vi "string to system.vi"(8 "error in":errorcluster, 10 "targets to load (all)":string[](array[string]), 11 "data":string) -> (0 "error out":errorcluster, 2 "system":T1)   [LabVIEW 2013, in "PLConfigurationSerializer.lvlib"]
uses:
  PLConfigurationSerializer.lvlib
  systems cluster.ctl
  system configuration/PL_System Configuration.lvclass
  targets cluster.ctl
  target configuration/PL_Target Configuration.lvclass
  engines cluster.ctl
  <vilib>/NI/Module Execution Interface/Engine Configuration/engine configuration.lvclass
  <vilib>/NI/Tag Bus Module Framework/module configuration/TBM module configuration.lvclass
  targetlist.ctl
  enginelist.ctl
  modulelist.ctl
  class discovery singleton methods.ctl
  <vilib>/NI/Tag Bus Module Framework/root configuration/TBM configuration.lvclass
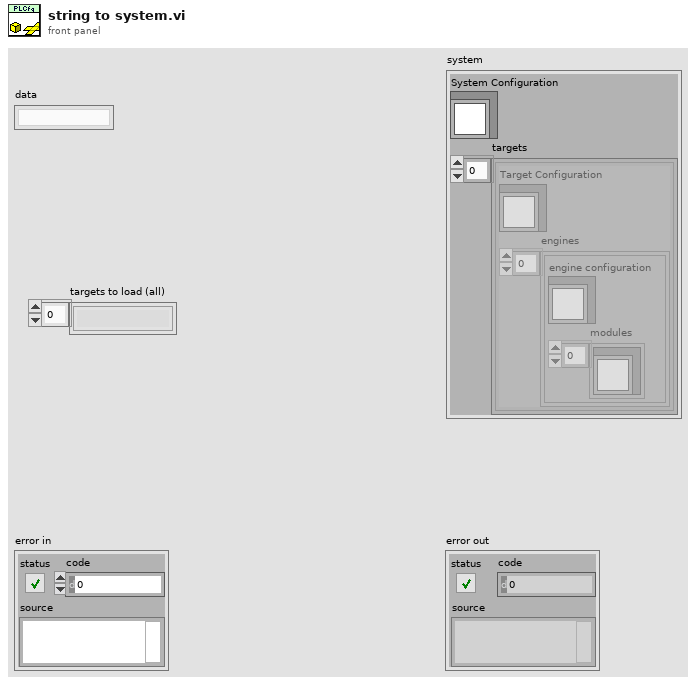
[diagram p1: front panel]
types:
  T1 = typedef "PLConfigurationSerializer.lvlib/systems cluster.ctl" = cluster{"System Configuration":refnum<class "PL_System Configuration.lvclass">, "targets":T2[]}
  T2 = typedef "PLConfigurationSerializer.lvlib/targets cluster.ctl" = cluster{"Target Configuration":refnum<class "PL_Target Configuration.lvclass">, "engines":T3[]}
  T3 = typedef "PLConfigurationSerializer.lvlib/engines cluster.ctl" = cluster{"engine configuration":refnum<class "engine configuration.lvclass">, "modules":refnum<class "TBM module configuration.lvclass">[]}
  T4 = typedef "PLConfigurationSerializer.lvlib/targetlist.ctl" = cluster{"name":string, "instanceid":string}
  T5 = typedef "PLConfigurationSerializer.lvlib/enginelist.ctl" = cluster{"engineid":string, "classname":string}
  T6 = typedef "PLConfigurationSerializer.lvlib/class discovery singleton methods.ctl" = enum16{"add search paths", "load class by name"}
  T7 = typedef "PLConfigurationSerializer.lvlib/modulelist.ctl" = cluster{"moduleid":string, "classname":string}
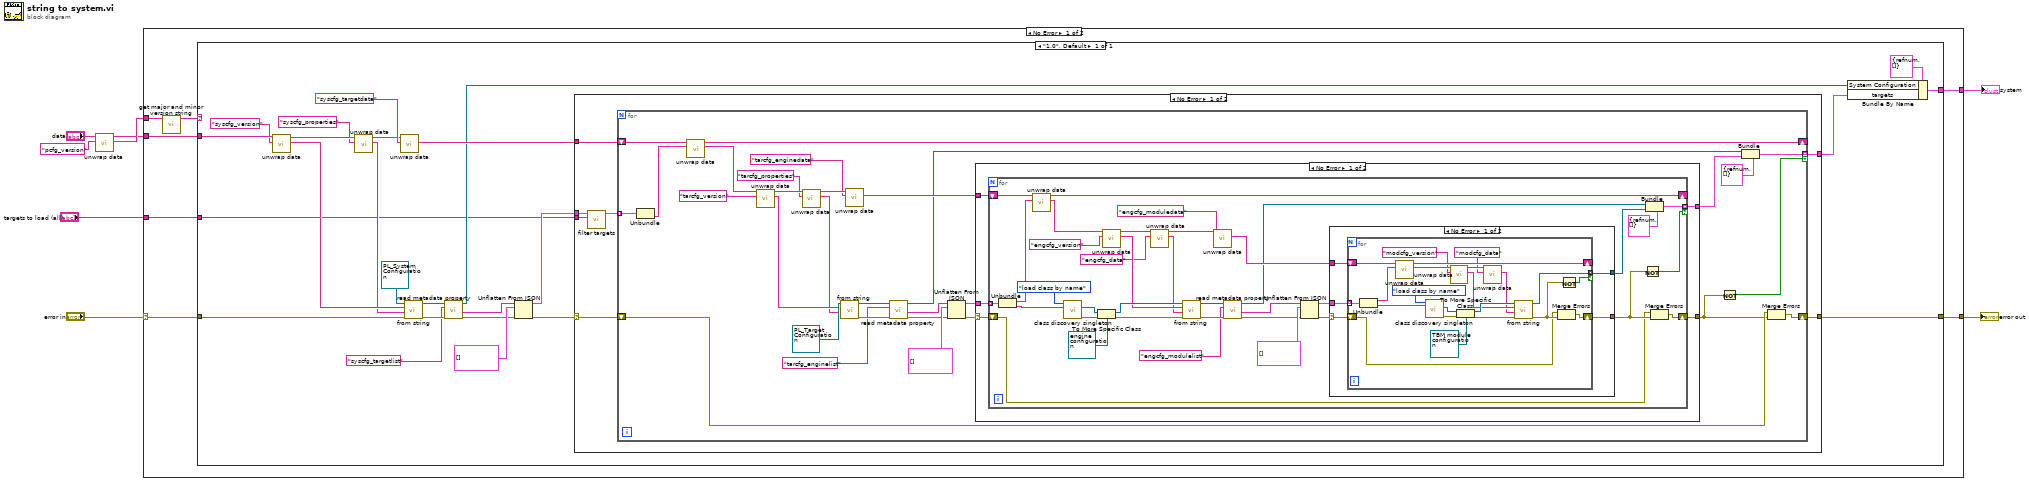
[diagram p0: block diagram]
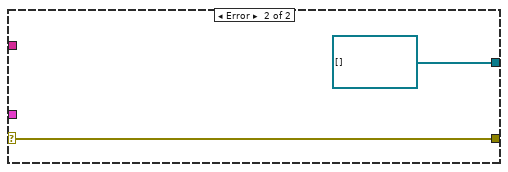
[diagram p2: hidden frame]
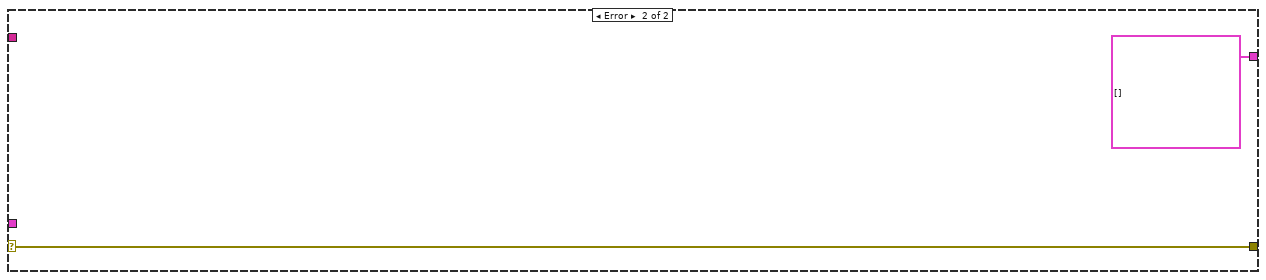
[diagram p3: hidden frame]
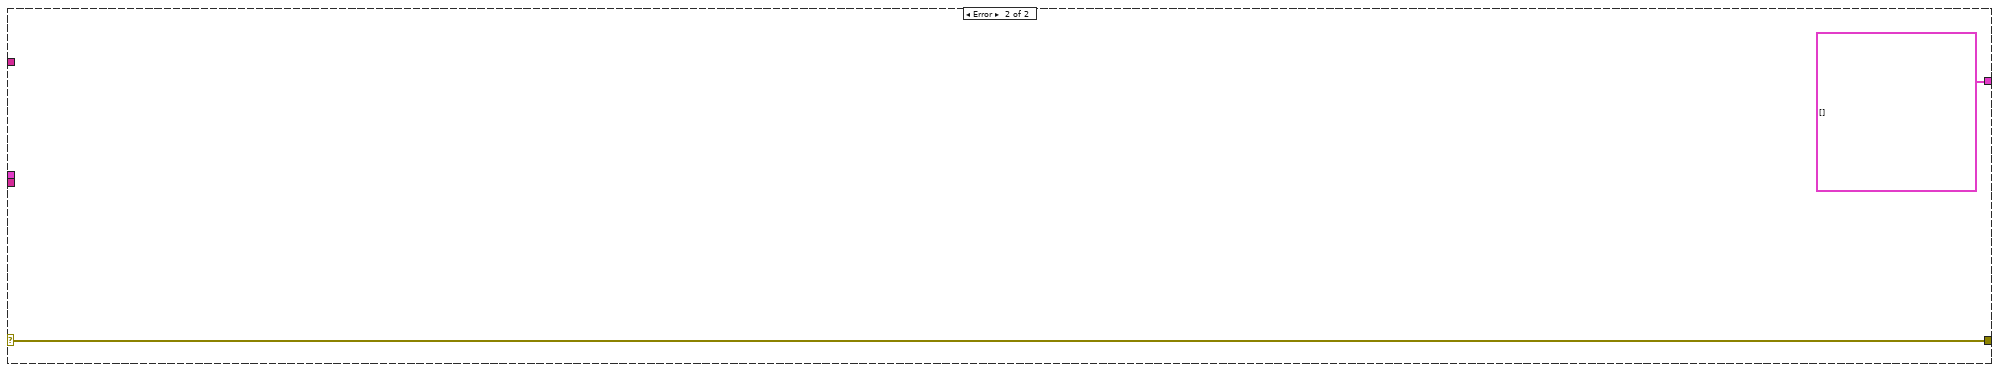
[diagram p4: hidden frame]
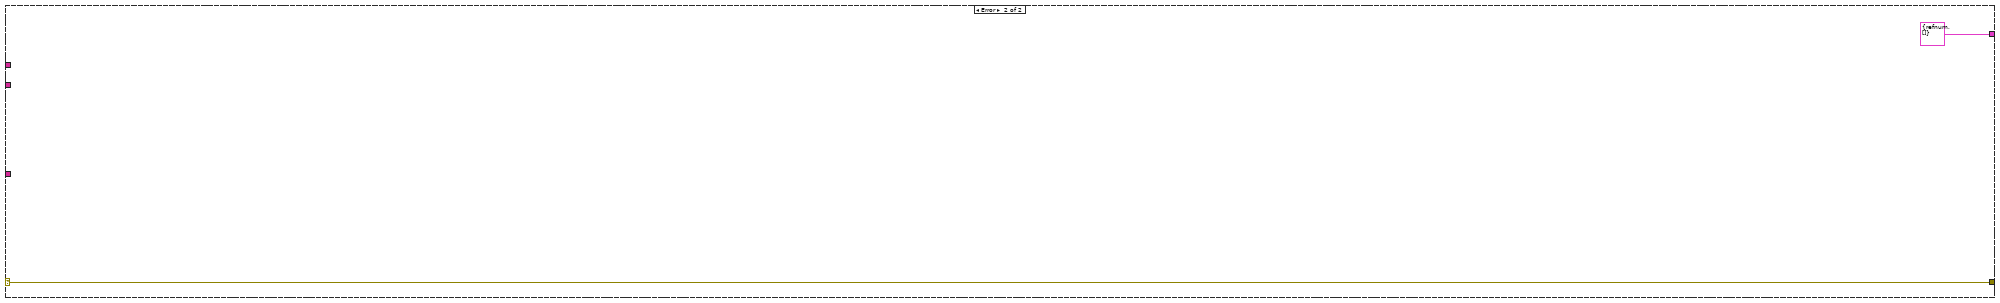
[diagram p5: hidden frame]
diagram:
  n1 = call <vilib>:"unwrap data.vi"("identifier"="pcfg_version" ("additional identifier"), "data to unwrap"="data") -> ("unwrapped data"=w7:string, "remaining string"=w6:string)  [unwired: 8 in]
  n2 = case shown="No Error" "error in" {
    selector: "error in" -> [w11 w153]
    tunnel: w6 -> [w15 _]
    tunnel: [w14 T1 {"System Configuration"=refnum, "targets"=[]} ("system")] -> w5
    tunnel: [w10 w153] -> w4
    tunnel: w7 -> [w13 _]
    tunnel: "targets to load (all)" -> [w9 _]
    frame No Error {
      n3 = call <vilib>:"get major and minor version string.vi"("full version"=w13) -> ("major.minor version"=w12:string)  [unwired: 10 in]
      n4 = case shown="\"1.0\", Default" w12 {
        tunnel: w15 -> [w40]
        tunnel: w11 -> [w36]
        tunnel: [w31] -> w14
        tunnel: [w29] -> w10
        tunnel: w9 -> [w17]
        frame "1.0", Default {
          n5 = call <vilib>:"unwrap data.vi"("identifier"="syscfg_version" ("additional identifier"), "data to unwrap"=w40) -> ("unwrapped data"=w34:string, "remaining string"=w39:string)  [unwired: 8 in]
          n6 = call <vilib>:"unwrap data.vi"("identifier"="syscfg_properties" ("additional identifier"), "data to unwrap"=w39) -> ("unwrapped data"=w33:string, "remaining string"=w20:string)  [unwired: 8 in]
          n7 = call <vilib>:"unwrap data.vi"("identifier"="syscfg_targetdata" ("additional identifier"), "data to unwrap"=w20) -> ("unwrapped data"=w28:string)  [unwired: 8 in, 1 out]
          n8 = call-dynamic "from string.vi"("error in"=w36, "data"=w33, "version"=w34, "configuration in"=refnum<class "PL_System Configuration.lvclass"> refnum) -> ("error out"=w22:errorcluster, "configuration out"=w25:refnum<class "PL_System Configuration.lvclass">)  [unwired: 6 in]
          n9 = call <vilib>:"read metadata property.vi"("error in"=w22, "key"="syscfg_targetlist" ("additional identifier"), "configuration in"=w25) -> ("error out"=w23:errorcluster, "value"=w19:string, "configuration out"=w24:refnum<class "PL_System Configuration.lvclass">)  [unwired: 5 in, 1 out]
          n10 = Unflatten From JSON(JSON string=w19, type and defaults=T4[] [], error in (no error)=w23) -> (value=w18:T4[], error out=w16:errorcluster)  [unwired: 4 in]
          n11 = case shown="No Error" w16 {
            selector: w16 -> [w41 w150]
            tunnel: [w47 w150] -> w29
            tunnel: w28 -> [w46 _]
            tunnel: [w45 T2[] []] -> w27
            tunnel: w18 -> [w44 _]
            tunnel: w17 -> [w42 _]
            frame No Error {
              n12 = call "filter targets.vi"("targets to load"=w42, "targets in"=w44) -> ("targets out"=w43:T4[])  [unwired: 9 in]
              n13 = for {
                shift-right: [w51] -> w47
                shift-left: w41 -> [w50]
                tunnel: w43 -> [w77] mode=indexing
                shift-right: [w75] -> _
                shift-left: w46 -> [w76]
                tunnel: [w73] -> w45 mode=indexing if=w48
                n14 = Unbundle(w77) -> ("instanceid"=w53:string)  [unwired: 1 out]
                n15 = call <vilib>:"unwrap data.vi"("identifier"=w53, "data to unwrap"=w76) -> ("unwrapped data"=w71:string, "remaining string"=w75:string)  [unwired: 8 in]
                n16 = call <vilib>:"unwrap data.vi"("identifier"="tarcfg_version" ("additional identifier"), "data to unwrap"=w71) -> ("unwrapped data"=w69:string, "remaining string"=w70:string)  [unwired: 8 in]
                n17 = call <vilib>:"unwrap data.vi"("identifier"="tarcfg_properties" ("additional identifier"), "data to unwrap"=w70) -> ("unwrapped data"=w68:string, "remaining string"=w65:string)  [unwired: 8 in]
                n18 = call-dynamic "from string.vi"("data"=w68, "version"=w69, "configuration in"=refnum<class "PL_Target Configuration.lvclass"> refnum ("configuration out")) -> ("error out"=w57:errorcluster, "configuration out"=w58:refnum<class "PL_Target Configuration.lvclass">)  [unwired: 7 in]
                n19 = call <vilib>:"unwrap data.vi"("identifier"="tarcfg_enginedata" ("additional identifier"), "data to unwrap"=w65) -> ("unwrapped data"=w60:string)  [unwired: 8 in, 1 out]
                n20 = call <vilib>:"read metadata property.vi"("error in"=w57, "key"="tarcfg_enginelist" ("additional identifier"), "configuration in"=w58) -> ("error out"=w56:errorcluster, "value"=w55:string, "configuration out"=w59:refnum<class "PL_Target Configuration.lvclass">)  [unwired: 5 in, 1 out]
                n21 = Unflatten From JSON(JSON string=w55, type and defaults=T5[] [], error in (no error)=w56) -> (value=w61:T5[], error out=w52:errorcluster)  [unwired: 4 in]
                n22 = case shown="No Error" w52 {
                  selector: w52 -> [w78 w149]
                  tunnel: [w82 T3[] []] -> w62
                  tunnel: w61 -> [w81 _]
                  tunnel: [w80 w149] -> w49
                  tunnel: w60 -> [w79 _]
                  frame No Error {
                    n23 = for {
                      tunnel: [w117] -> w82 mode=indexing if=w87
                      shift-right: [w86] -> w80
                      shift-left: w78 -> [w84]
                      tunnel: w81 -> [w116] mode=indexing
                      shift-right: [w114] -> _
                      shift-left: w79 -> [w115]
                      n24 = Unbundle(w116) -> ("engineid"=w113:string, "classname"=w89:string)
                      n25 = call <vilib>:"unwrap data.vi"("identifier"=w113, "data to unwrap"=w115) -> ("unwrapped data"=w109:string, "remaining string"=w114:string)  [unwired: 8 in]
                      n26 = call "class discovery singleton.vi"("Class Name"=w89, "method"=class_discovery_singleton_methods."load class by name") -> ("error out"=w91:errorcluster, "LabVIEW Object"=w90:refnum<class>)  [unwired: 8 in]
                      n27 = To More Specific Class(target class=refnum<class "engine configuration.lvclass"> refnum ("engine configuration"), reference=w90, error in=w91) -> (specific class reference=w110:refnum<class "engine configuration.lvclass">, error out=w111:errorcluster)
                      n28 = call <vilib>:"unwrap data.vi"("identifier"="engcfg_version" ("additional identifier"), "data to unwrap"=w109) -> ("unwrapped data"=w106:string, "remaining string"=w107:string)  [unwired: 8 in]
                      n29 = call <vilib>:"unwrap data.vi"("identifier"="engcfg_data" ("additional identifier"), "data to unwrap"=w107) -> ("unwrapped data"=w104:string, "remaining string"=w103:string)  [unwired: 8 in]
                      n30 = call-dynamic "from string.vi"("error in"=w111, "data"=w104, "version"=w106, "engine configuration in"=w110) -> ("error out"=w94:errorcluster, "engine configuration out"=w95:refnum<class "engine configuration.lvclass">)  [unwired: 6 in]
                      n31 = call <vilib>:"unwrap data.vi"("identifier"="engcfg_moduledata" ("additional identifier"), "data to unwrap"=w103) -> ("unwrapped data"=w100:string)  [unwired: 8 in, 1 out]
                      n32 = call <vilib>:"read metadata property.vi"("error in"=w94, "key"="engcfg_modulelist" ("additional identifier"), "configuration in"=w95) -> ("error out"=w97:errorcluster, "value"=w92:string, "configuration out"=w96:refnum<class "engine configuration.lvclass">)  [unwired: 5 in, 1 out]
                      n33 = Unflatten From JSON(JSON string=w92, type and defaults=T7[] [], error in (no error)=w97) -> (value=w99:T7[], error out=w83:errorcluster)  [unwired: 4 in]
                      n34 = case shown="No Error" w83 {
                        selector: w83 -> [w119 w146]
                        tunnel: w100 -> [w123 _]
                        tunnel: w99 -> [w122 _]
                        tunnel: [w121 refnum<class "TBM module configuration.lvclass">[] []] -> w98
                        tunnel: [w120 w146] -> w85
                        frame No Error {
                          n35 = for {
                            shift-right: [w125] -> w120
                            shift-left: w119 -> [w124]
                            shift-right: [w142] -> _
                            shift-left: w123 -> [w144]
                            tunnel: w122 -> [w145] mode=indexing
                            tunnel: [w137] -> w121 mode=indexing if=w127
                            n36 = Unbundle(w145) -> ("moduleid"=w143:string, "classname"=w128:string)
                            n37 = call <vilib>:"unwrap data.vi"("identifier"=w143, "data to unwrap"=w144) -> ("unwrapped data"=w140:string, "remaining string"=w142:string)  [unwired: 8 in]
                            n38 = call "class discovery singleton.vi"("Class Name"=w128, "method"=class_discovery_singleton_methods."load class by name") -> ("error out"=w130:errorcluster, "LabVIEW Object"=w129:refnum<class>)  [unwired: 8 in]
                            n39 = call <vilib>:"unwrap data.vi"("identifier"="modcfg_version" ("additional identifier"), "data to unwrap"=w140) -> ("unwrapped data"=w136:string, "remaining string"=w135:string)  [unwired: 8 in]
                            n40 = To More Specific Class(target class=refnum<class "TBM module configuration.lvclass"> refnum ("module configuration"), reference=w129, error in=w130) -> (specific class reference=w138:refnum<class "TBM module configuration.lvclass">, error out=w139:errorcluster)
                            n41 = call <vilib>:"unwrap data.vi"("identifier"="modcfg_data" ("additional identifier"), "data to unwrap"=w135) -> ("unwrapped data"=w134:string)  [unwired: 8 in, 1 out]
                            n42 = call-dynamic "from string.vi"("error in"=w139, "data"=w134, "version"=w136, "module configuration in"=w138) -> ("error out"=w126:errorcluster, "module configuration out"=w137:refnum<class "TBM module configuration.lvclass">)  [unwired: 6 in]
                            n43 = Merge Errors(w124, w126) -> (w125:errorcluster)
                            n44 = Not(x=w126) -> (.not. x?=w127:bool)
                          }
                        }
                        frame Error {
                        }
                      }
                      n45 = Not(x=w85) -> (.not. x?=w87:bool)
                      n46 = Bundle(cluster=T3 {"engine configuration"=refnum, "modules"=[]} ("engines cluster"), "engine configuration"=w96, "modules"=w98) -> (w117:T3)
                      n47 = Merge Errors(w84, w85) -> (w86:errorcluster)
                    }
                  }
                  frame Error {
                  }
                }
                n48 = Not(x=w49) -> (.not. x?=w48:bool)
                n49 = Bundle(cluster=T2 {"Target Configuration"=refnum, "engines"=[]} ("targets cluster"), "Target Configuration"=w59, "engines"=w62) -> (w73:T2)
                n50 = Merge Errors(w50, w49) -> (w51:errorcluster)
              }
            }
            frame Error {
            }
          }
          n51 = Bundle By Name(cluster=T1 {"System Configuration"=refnum, "targets"=[]} ("system"), "System Configuration"=w24, "targets"=w27) -> (w31:T1)
        }
      }
    }
    frame Error {
    }
  }
  "system" <- w5
  "error out" <- w4
